vi "FTW-Actor-Log-Event.vi"(0 "FTW Actor Instance":refnum<class "FTW-ActorInstance.lvclass">, 5 "Event Type":string, 7 "Event Data":string, 9 "Source (unwired for identity)":string="Identity", 11 "error in":errorcluster) -> (4 "FTW Actor Instance out":refnum<class "FTW-ActorInstance.lvclass">, 6 "Serialized Event":string, 15 "error out":errorcluster)   [LabVIEW 2015, in "FTW-ActorInstance.lvclass"]
uses:
  FTW-ActorInstance.lvclass
  FTW-ActorInstance.lvclass/FTW-ActorInstance.ctl
  EventLogger/FTW-Logger.lvclass
panel:
  # "Inputs"
  # "Outputs"
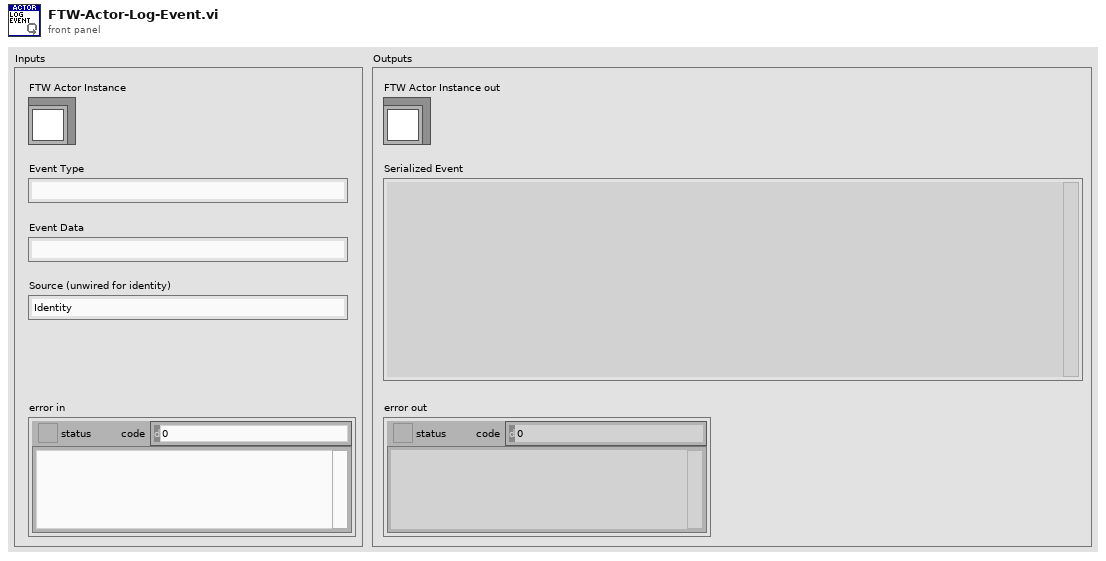
[diagram p1: front panel]
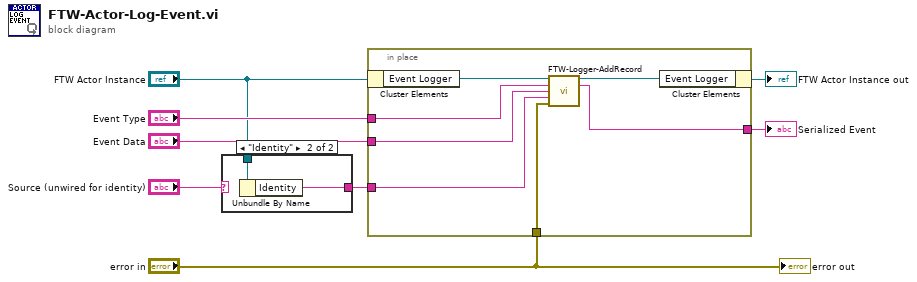
[diagram p0: block diagram]
diagram:
  n1 = case shown="\"Identity\"" "Source (unwired for identity)" {
    selector: "Source (unwired for identity)" -> [w9 _]
    tunnel: "FTW Actor Instance" -> [_ w11]
    tunnel: [w9 w10] -> w2
    frame Default {
    }
    frame "Identity" {
      n2 = Unbundle By Name(w11) -> ("Identity"=w10:string)
    }
  }
  n3 = in-place {
    in-place-border: "error in" -> [w18]
    in-place-border: [w15] -> w7
    in-place-border: "Event Type" -> [w14]
    in-place-border: "Event Data" -> [w13]
    in-place-border: w2 -> [w12]
    n4 = in-place-cluster #1("FTW Actor Instance") -> ("Event Logger"=w17:refnum<class "FTW-Logger.lvclass">)
    n5 = call "FTW-Logger-AddRecord.vi"("FTW Logger Connector"=w17, "Event Type"=w14, "Event Data"=w13, "Source (unwired for call chain)"=w12, "error in"=w18) -> ("FTW Logger Connector out"=w16:refnum<class "FTW-Logger.lvclass">, "Serialized Event"=w15:string)  [unwired: 8 in, 1 out]
    n6 = in-place-cluster #1("Event Logger"=w16) -> (→"FTW Actor Instance out":refnum<class "FTW-ActorInstance.lvclass">)
  }
  "Serialized Event" <- w7
  "error out" <- "error in"
